vi "Actor Core.vi"(8 "error in":errorcluster, 11 "TopButton In":refnum<class "TopButton.lvclass">) -> (0 "error out":errorcluster, 3 "Actor out":refnum<class "Actor.lvclass">)   [LabVIEW 2017, in "TopButton.lvlib" / "TopButton.lvclass"]
uses:
  <vilib>/gpm_packages/TestSystem/Views/TopButton/TopButton/TopButton.lvclass
  C:/Program Files/National Instruments/LabVIEW 2017/vi.lib/gpm_packages/@cs/mva-viewable/Source/ActorEvents/IEventAggregator/IEventAggregator.lvclass
  C:/Program Files/National Instruments/LabVIEW 2017/vi.lib/gpm_packages/@cs/mva-viewable/Source/IViewable/IViewable/IViewable.lvclass
  <vilib>/ActorFramework/Actor/Actor.lvclass
  <vilib>/event_ctls.llb/lveventtype.ctl
  <vilib>/gpm_packages/@cs/mva-viewable/Source/IViewable/IViewable/IViewable.lvclass
  <vilib>/gpm_packages/@cs/mva-viewable/Source/ActorEvents/IEventAggregator/IEventAggregator.lvclass
panel:
  in  "Serial  Number Input":string
  in  "SFC":bool
  out "CleTime":dbl
  out "Slot":T1(ring)
  out "Tested":i32
  out "Failed":i32
  out "Passed":i32
  in  "Stop":bool
  in  "Pause":bool
  in  "Start":bool
  out "Result":string
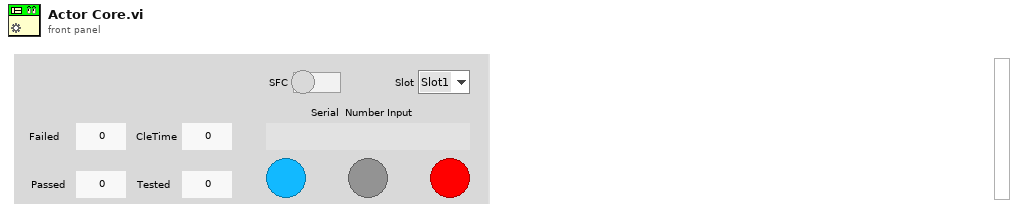
[diagram p1: front panel]
types:
  T1 = enum16{"Slot1", "Slot2", "Slot3", "Slot4", "Slot5", "Slot6", "Slot7", "Slot8", "Slot9", "Slot10", "Slot11", "Slot12", "Slot13", "Slot14", "Slot15", "Slot16", "Slot17", "Slot18", "Slot19", "Slot20", "Slot21", "Slot22", "Slot23", "Slot24", "Slot25", "Slot26", "Slot27", "Slot28", "Slot29", "Slot30", "Slot31", "Slot32"}
  T2 = typedef "lveventtype.ctl" = enum32{"Null", "Timeout", "Annotation Menu Selection", "Annotation Menu Selection?", "App Instance Close", "App Instance Close?", "Autoscale Range Change", "Bookmark Info Change", "Cell Edit", "Cell Edit?", "Cursor Grab", "Cursor Grab?", "Cursor Menu Selection", "Cursor Menu Selection?", "Cursor Move", "Cursor Release", "Data Change", "Direction Change", "Display State Change", "Drag Ended", "Drag Enter", "Drag Leave", "Drag Over", "Drag Source Update", "Drag Starting", "Drag Starting?", "Drop", "Exec State Change", "Key Down", "Key Down?", "Key Repeat", "Key Repeat?", "Key Up", "Listbox Double Click", "Menu Activation?", "Menu Selection (App)", "Menu Selection? (App)", "Menu Selection (User)", "Mouse Down", "Mouse Down?", "Mouse Enter", "Mouse Leave", "Mouse Move", "Mouse Up", "Mouse Wheel", "NI Security User Change (App)", "Pane Size", "Panel Close", "Panel Close?", "Panel Resize", "Plot Attribute Change", "Scale Range Change", "Shortcut Menu Activation?", "Shortcut Menu Selection (App)", "Shortcut Menu Selection? (App)", "Shortcut Menu Selection (User)", "Tree Double Click", "Tree Drag", "Tree Drag?", "Tree Drop", "Tree Drop?", "Tree Item Close", "Tree Item Close?", "Tree Item Open", "Tree Item Open?", "User Event", "Value Change"}
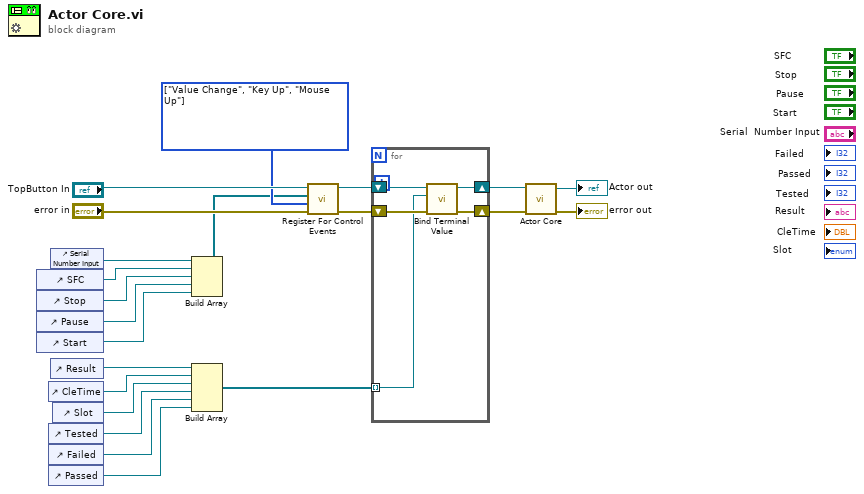
[diagram p0: block diagram]
diagram:
  w18 = T2[] [enum."Value Change", enum."Key Up", enum."Mouse Up"] items=["Null", "Timeout", "Annotation Menu Selection", "Annotation Menu Selection?", "App Instance Close", "App Instance Close?", "Autoscale Range Change", "Bookmark Info Change", "Cell Edit", "Cell Edit?", "Cursor Grab", "Cursor Grab?", "Cursor Menu Selection", "Cursor Menu Selection?", "Cursor Move", "Cursor Release", "Data Change", "Direction Change", "Display State Change", "Drag Ended", "Drag Enter", "Drag Leave", "Drag Over", "Drag Source Update", "Drag Starting", "Drag Starting?", "Drop", "Exec State Change", "Key Down", "Key Down?", "Key Repeat", "Key Repeat?", "Key Up", "Listbox Double Click", "Menu Activation?", "Menu Selection (App)", "Menu Selection? (App)", "Menu Selection (User)", "Mouse Down", "Mouse Down?", "Mouse Enter", "Mouse Leave", "Mouse Move", "Mouse Up", "Mouse Wheel", "NI Security User Change (App)", "Pane Size", "Panel Close", "Panel Close?", "Panel Resize", "Plot Attribute Change", "Scale Range Change", "Shortcut Menu Activation?", "Shortcut Menu Selection (App)", "Shortcut Menu Selection? (App)", "Shortcut Menu Selection (User)", "Tree Double Click", "Tree Drag", "Tree Drag?", "Tree Drop", "Tree Drop?", "Tree Item Close", "Tree Item Close?", "Tree Item Open", "Tree Item Open?", "User Event", "Value Change"] ("Registration Types")
  n1 = control-ref of="SFC"() -> (w8:refnum<vi>)
  n2 = control-ref of="Stop"() -> (w16:refnum<vi>)
  n3 = control-ref of="Pause"() -> (w15:refnum<vi>)
  n4 = control-ref of="Start"() -> (w14:refnum<vi>)
  n5 = control-ref of="CleTime"() -> (w6:refnum<vi>)
  n6 = control-ref of="Tested"() -> (w4:refnum<vi>)
  n7 = control-ref of="Failed"() -> (w3:refnum<vi>)
  n8 = control-ref of="Passed"() -> (w2:refnum<vi>)
  n9 = control-ref of="Serial  Number Input"() -> (w17:refnum<vi>)
  n10 = control-ref of="Result"() -> (w7:refnum<vi>)
  n11 = control-ref of="Slot"() -> (w5:refnum<vi>)
  n12 = Build Array(w17, w8, w16, w15, w14) -> (w13:refnum<vi>[])
  n13 = Build Array(w7, w6, w5, w4, w3, w2) -> (w1:refnum<vi>[])
  n14 = call <vilib>:"Register For Control Events.vi"("error in (no error)"="error in", "Registration Types"=w18, "Control Refnums"=w13, "IEventAggregator In"="TopButton In") -> ("error out"=w9:errorcluster, "IEventAggregator Out"=w12:refnum<class "TopButton.lvclass">)  [unwired: 6 in]
  n15 = for {
    tunnel: w1 -> [w23] mode=indexing
    shift-right: [w26] -> w11
    shift-left: w12 -> [w27]
    shift-right: [w25] -> w10
    shift-left: w9 -> [w24]
    n16 = call <vilib>:"Bind Terminal Value.vi"("error in (no error)"=w24, "Ctl Refnum"=w23, "IViewable in"=w27) -> ("error out"=w25:errorcluster, "IViewable out"=w26:refnum<class "TopButton.lvclass">)  [unwired: 7 in]
  }
  n17 = call-parent "Actor Core.vi"("error in"=w10, "IViewable In"=w11) -> ("error out"=→"error out":errorcluster, "Actor out"=→"Actor out":refnum<class "Actor.lvclass">)  [unwired: 8 in]
